vi "UnboxString.vi"(10 "String in":refnum<class "String.lvclass">) -> (2 "String":string)   [LabVIEW 2013, in "LapDog.Collections.v1.Common.lvlib" / "String.lvclass"]
uses:
  String.lvclass
  String.lvclass/String.ctl
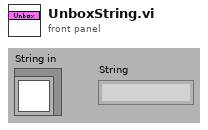
[diagram p1: front panel]
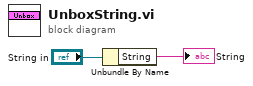
[diagram p0: block diagram]
diagram:
  n1 = Unbundle By Name("String in") -> ("String"=→"String":string)
